vi "RT_WavaFrequencyMeasurement.vi"() -> ()   [LabVIEW 2019]
uses:
  <vilib>/FPGAPlugInAG/ELVIS III/niLvFpga_Open_ELVIS III.vi
  <vilib>/rvi/interface/common/dynamic/niFpgaDynamicAddResources.vi
  <vilib>/myRIO/Common/Instrument Driver Framework/Utilities/vis/FPGA Ref Manager.vi
  <vilib>/Utility/error.llb/Error Cluster From Error Code.vi
  <vilib>/myRIO/Common/Instrument Driver Framework/Utilities/vis/Ref Counter.vi
  <vilib>/rvi/errors/niLvFpgaAdjustHostInterfaceError.vi
  <vilib>/FPGAPlugInAG/Dynamic/niLvFpga_Close_Dynamic.vi
  <vilib>/rvi/interface/nirviOpenFPGA/nirviOpenFPGA.xnode
  FPGA Bitfiles/measurementpwmfr_FPGATarget_WavaFrequencyMea_gxgqskmLuas.lvbitx
  WavaFrequencyMeasurement2.vi
  <vilib>/rvi/interface/nirviReadWriteControl/nirviReadWriteControl.xnode
  <vilib>/rvi/interface/nirviCloseFPGA/nirviCloseFPGA.xnode
  <vilib>/myRIO/Instrument Drivers/Utilities/Utilities.lvlib
  NiFpgaLv.dll
  <vilib>/rvi/interface/Simulation/niFpgaSimulationCallBeginRW.vi
panel:
  out "error out":errorcluster
  in  "Stop":bool
  out "波形图表":dbl(graph)
  out "频率":dbl format="%#_14g"
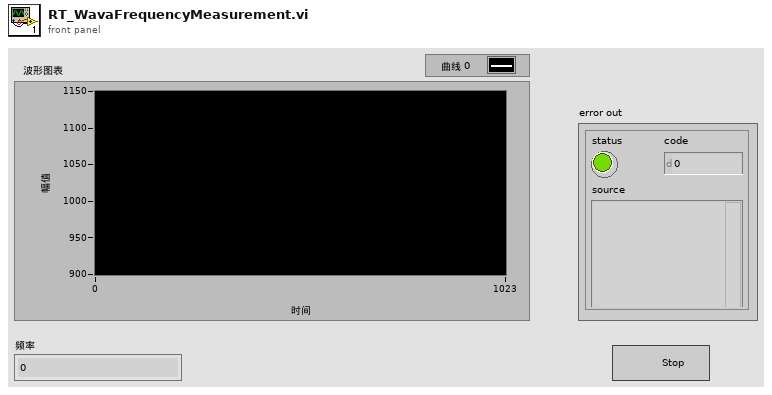
[diagram p1: front panel]
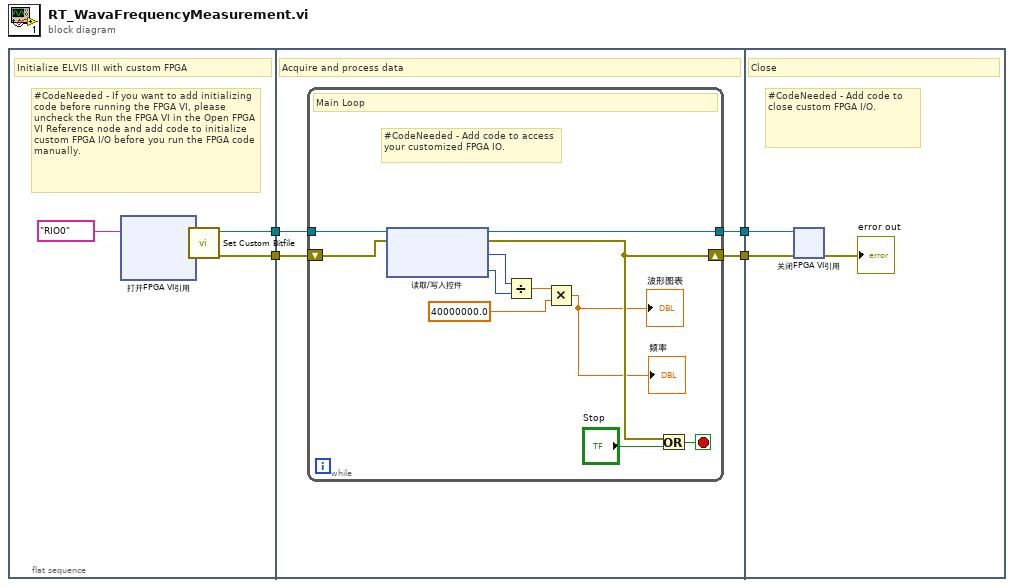
[diagram p0: block diagram]
diagram:
  n1 = flat-sequence {
    tunnel: [w6] -> w4
    tunnel: [w7] -> w3
    tunnel: w4 -> [w13]
    tunnel: w3 -> [w12]
    tunnel: [w11] -> w2
    tunnel: [w10] -> w1
    tunnel: w2 -> [w27]
    tunnel: w1 -> [w26]
    frame #0 {
      # "#CodeNeeded - If you want to add initializing code before running the FPGA VI, please uncheck the Run the FPGA VI in the Open FPGA VI Reference node and add code to initialize custom FPGA I/O before you run the FPGA code manually."
      # "Initialize ELVIS III with custom FPGA"
      n2 = xnode "打开FPGA VI引用"("资源名称"=tag "RIO0" ("resource name")) -> ("FPGA VI引用输出"=w8:refnum<k20>, "错误输出"=w9:errorcluster)  [unwired: 1 in]
      n3 = call <vilib>:"Set Custom Bitfile.vi"("error in (no error)"=w9, "Custom FPGA Reference In"=w8) -> ("error out"=w6:errorcluster, "Custom FPGA Reference Out"=w7:refnum<k20>)  [unwired: 8 in]
    }
    frame #1 {
      # "Acquire and process data"
      n4 = while {
        tunnel: w12 -> [w22]
        tunnel: [w21] -> w11
        shift-right: [w19] -> w10
        shift-left: w13 -> [w20]
        stop <- w23 stop-if-true
        # "#CodeNeeded - Add code to access your customized FPGA IO."
        # "Main Loop"
        n5 = xnode "读取/写入控件"("FPGA VI引用输入"=w22, "错误输入"=w20) -> ("FPGA VI引用输出"=w21:refnum<k20>, "错误输出"=w19:errorcluster, "被测信号个数 2"=w15:u32, "时钟信号个数 2"=w14:u32)
        n6 = Divide(x=w15, y=w14) -> (x/y=w18:dbl)
        n7 = Multiply(x=w18, y=40000000.0) -> (x*y=→"波形图表" →"频率":dbl)
        n8 = Or(x=w19, y="Stop") -> (x .or. y?=w23:bool)
      }
    }
    frame #2 {
      # "#CodeNeeded - Add code to close custom FPGA I/O."
      # "Close"
      n9 = xnode "关闭FPGA VI引用"("FPGA VI引用输入"=w27, "错误输入"=w26) -> ("错误输出"=→"error out":errorcluster)
    }
  }
